vi "oax_Config TIO and DSA Channel (Single Shot).vi"(0 "master":T1={"DSA Device"="", "Channels"={"enable ch0"=FALSE, "enable ch1"=FALSE, "enable ch2"=FALSE, "enable ch3"=FALSE, "enable ch4"=FALSE, "enable ch5"=FALSE, "enable ch6"=FALSE, "enable ch7"=FALSE}, "Channel Names"={"ch0 string"="", "ch1 string"="", "ch2 string"="", "ch3 string"="", "ch4 string"="", "ch5 string"="", "ch6 string"="", "ch7 string"=""}, "Coupling"={"coupling ch0"=FALSE, "coupling ch1"=FALSE, "coupling ch2"=FALSE, "coupling ch3"=FALSE, "coupling ch4"=FALSE, "coupling ch5"=FALSE, "coupling ch6"=FALSE, "coupling ch7"=FALSE}, "IEPE"={"ICP ch0"=FALSE, "ICP ch0"=FALSE, "ICP ch0"=FALSE, "ICP ch0"=FALSE, "ICP ch0"=FALSE, "ICP ch0"=FALSE, "ICP ch0"=FALSE, "ICP ch0"=FALSE}, "Ch. Sensitivity\n[mV/EU]"={"ch0 sensitivity"=1000.0, "ch1 sensitivity"=1000.0, "ch2 sensitivity"=1000.0, "ch3 sensitivity"=1000.0, "ch4 sensitivity"=1000.0, "ch5 sensitivity"=1000.0, "ch6 sensitivity"=1000.0, "ch7 sensitivity"=1000.0}, "Engineering\nUnits"={"Engineering\nUnits"=0, "Engineering\nUnits"=0, "Engineering\nUnits"=0, "Engineering\nUnits"=0, "Engineering\nUnits"=0, "Engineering\nUnits"=0, "Engineering\nUnits"=0, "Engineering\nUnits"=0}, "Custom\nLabel"={"Custom Label"="", "Custom Label"="", "Custom Label"="", "Custom Label"="", "Custom Label"="", "Custom Label"="", "Custom Label"="", "Custom Label"=""}, "dB reference\n[EU]"={"dB reference [EU]"=1.0, "dB reference [EU]"=1.0, "dB reference [EU]"=1.0, "dB reference [EU]"=1.0, "dB reference [EU]"=1.0, "dB reference [EU]"=1.0, "dB reference [EU]"=1.0, "dB reference [EU]"=1.0}, "pregain\n[dB]"={"pregain [dB]"=0.0, "pregain [dB]"=0.0, "pregain [dB]"=0.0, "pregain [dB]"=0.0, "pregain [dB]"=0.0, "pregain [dB]"=0.0, "pregain [dB]"=0.0, "pregain [dB]"=0.0}, "Weighting\nFilter"={"Weighting Filter"=0, "Weighting Filter"=0, "Weighting Filter"=0, "Weighting Filter"=0, "Weighting Filter"=0, "Weighting Filter"=0, "Weighting Filter"=0, "Weighting Filter"=0}, "max value"=10.0, "min value"=0.0, "enable EAR?"=FALSE} {"min value" format="%0.2f"; "max value" format="%0.2f"; "Weighting\nFilter"."Weighting Filter" items=["Linear", "A-weighting", "B-weighting", "C-weighting", "ITU-R 468-4", "Dolby", "CCITT", "C-message"]; "Weighting\nFilter"."Weighting Filter" items=["Linear", "A-weighting", "B-weighting", "C-weighting", "ITU-R 468-4", "Dolby", "CCITT", "C-message"]; "Weighting\nFilter"."Weighting Filter" items=["Linear", "A-weighting", "B-weighting", "C-weighting", "ITU-R 468-4", "Dolby", "CCITT", "C-message"]; "Weighting\nFilter"."Weighting Filter" items=["Linear", "A-weighting", "B-weighting", "C-weighting", "ITU-R 468-4", "Dolby", "CCITT", "C-message"]; "Weighting\nFilter"."Weighting Filter" items=["Linear", "A-weighting", "B-weighting", "C-weighting", "ITU-R 468-4", "Dolby", "CCITT", "C-message"]; "Weighting\nFilter"."Weighting Filter" items=["Linear", "A-weighting", "B-weighting", "C-weighting", "ITU-R 468-4", "Dolby", "CCITT", "C-message"]; "Weighting\nFilter"."Weighting Filter" items=["Linear", "A-weighting", "B-weighting", "C-weighting", "ITU-R 468-4", "Dolby", "CCITT", "C-message"]; "Weighting\nFilter"."Weighting Filter" items=["Linear", "A-weighting", "B-weighting", "C-weighting", "ITU-R 468-4", "Dolby", "CCITT", "C-message"]; "pregain\n[dB]"."pregain [dB]" format="%.2f"; "pregain\n[dB]"."pregain [dB]" format="%.2f"; "pregain\n[dB]"."pregain [dB]" format="%.2f"; "pregain\n[dB]"."pregain [dB]" format="%.2f"; "pregain\n[dB]"."pregain [dB]" format="%.2f"; "pregain\n[dB]"."pregain [dB]" format="%.2f"; "pregain\n[dB]"."pregain [dB]" format="%.2f"; "pregain\n[dB]"."pregain [dB]" format="%.2f"; "dB reference\n[EU]"."dB reference [EU]" format="%^.1e"; "dB reference\n[EU]"."dB reference [EU]" format="%^.1e"; "dB reference\n[EU]"."dB reference [EU]" format="%^.1e"; "dB reference\n[EU]"."dB reference [EU]" format="%^.1e"; "dB reference\n[EU]"."dB reference [EU]" format="%^.1e"; "dB reference\n[EU]"."dB reference [EU]" format="%^.1e"; "dB reference\n[EU]"."dB reference [EU]" format="%^.1e"; "dB reference\n[EU]"."dB reference [EU]" format="%^.1e"; "Engineering\nUnits"."Engineering\nUnits" items=["custom..."=0, "V"=1, "A"=21, "Pa"=2, "N"=20, "g"=3, "m/s^2"=4, "m/s"=5, "m"=6, "mm/s"=12, "mm"=13, "microns/s"=14, "microns"=15, "in/s^2"=7, "in/s"=8, "in"=9, "mils/s"=10, "mils"=11, "rad/s^2"=16, "rad/s"=17, "rad"=18, "strain"=19]; "Engineering\nUnits"."Engineering\nUnits" items=["custom..."=0, "V"=1, "A"=21, "Pa"=2, "N"=20, "g"=3, "m/s^2"=4, "m/s"=5, "m"=6, "mm/s"=12, "mm"=13, "microns/s"=14, "microns"=15, "in/s^2"=7, "in/s"=8, "in"=9, "mils/s"=10, "mils"=11, "rad/s^2"=16, "rad/s"=17, "rad"=18, "strain"=19]; "Engineering\nUnits"."Engineering\nUnits" items=["custom..."=0, "V"=1, "A"=21, "Pa"=2, "N"=20, "g"=3, "m/s^2"=4, "m/s"=5, "m"=6, "mm/s"=12, "mm"=13, "microns/s"=14, "microns"=15, "in/s^2"=7, "in/s"=8, "in"=9, "mils/s"=10, "mils"=11, "rad/s^2"=16, "rad/s"=17, "rad"=18, "strain"=19]; "Engineering\nUnits"."Engineering\nUnits" items=["custom..."=0, "V"=1, "A"=21, "Pa"=2, "N"=20, "g"=3, "m/s^2"=4, "m/s"=5, "m"=6, "mm/s"=12, "mm"=13, "microns/s"=14, "microns"=15, "in/s^2"=7, "in/s"=8, "in"=9, "mils/s"=10, "mils"=11, "rad/s^2"=16, "rad/s"=17, "rad"=18, "strain"=19]; "Engineering\nUnits"."Engineering\nUnits" items=["custom..."=0, "V"=1, "A"=21, "Pa"=2, "N"=20, "g"=3, "m/s^2"=4, "m/s"=5, "m"=6, "mm/s"=12, "mm"=13, "microns/s"=14, "microns"=15, "in/s^2"=7, "in/s"=8, "in"=9, "mils/s"=10, "mils"=11, "rad/s^2"=16, "rad/s"=17, "rad"=18, "strain"=19]; "Engineering\nUnits"."Engineering\nUnits" items=["custom..."=0, "V"=1, "A"=21, "Pa"=2, "N"=20, "g"=3, "m/s^2"=4, "m/s"=5, "m"=6, "mm/s"=12, "mm"=13, "microns/s"=14, "microns"=15, "in/s^2"=7, "in/s"=8, "in"=9, "mils/s"=10, "mils"=11, "rad/s^2"=16, "rad/s"=17, "rad"=18, "strain"=19]; "Engineering\nUnits"."Engineering\nUnits" items=["custom..."=0, "V"=1, "A"=21, "Pa"=2, "N"=20, "g"=3, "m/s^2"=4, "m/s"=5, "m"=6, "mm/s"=12, "mm"=13, "microns/s"=14, "microns"=15, "in/s^2"=7, "in/s"=8, "in"=9, "mils/s"=10, "mils"=11, "rad/s^2"=16, "rad/s"=17, "rad"=18, "strain"=19]; "Engineering\nUnits"."Engineering\nUnits" items=["custom..."=0, "V"=1, "A"=21, "Pa"=2, "N"=20, "g"=3, "m/s^2"=4, "m/s"=5, "m"=6, "mm/s"=12, "mm"=13, "microns/s"=14, "microns"=15, "in/s^2"=7, "in/s"=8, "in"=9, "mils/s"=10, "mils"=11, "rad/s^2"=16, "rad/s"=17, "rad"=18, "strain"=19]; "Ch. Sensitivity\n[mV/EU]"."ch7 sensitivity" format="%.2f"; "Ch. Sensitivity\n[mV/EU]"."ch6 sensitivity" format="%.2f"; "Ch. Sensitivity\n[mV/EU]"."ch5 sensitivity" format="%.2f"; "Ch. Sensitivity\n[mV/EU]"."ch4 sensitivity" format="%.2f"; "Ch. Sensitivity\n[mV/EU]"."ch3 sensitivity" format="%.2f"; "Ch. Sensitivity\n[mV/EU]"."ch2 sensitivity" format="%.2f"; "Ch. Sensitivity\n[mV/EU]"."ch1 sensitivity" format="%.2f"; "Ch. Sensitivity\n[mV/EU]"."ch0 sensitivity" format="%.2f"}, 1 "samples per channel":u32, 2 "sample rate [samples/s]":dbl, 5 "Counter(s)":tag, 9 "PFI line (Gate)":tag, 11 "error out":errorcluster, 12 "Tacho Pulse Edge":i32, 13 "Slave Slot Number":i32(ring) caption="PXI Slot Number" items=["Slot 3", "Slot 4", "Slot 5", "Slot 6", "Slot 7", "Slot 8", "Slot 9", "Slot 10", "Slot 11", "Slot 12", "Slot 13", "Slot 14", "Slot 15", "Slot 16"], 14 "DSA device type":u16(ring) items=["447x", "446x"]) -> (4 "DSA task out":refnum<k21>, 6 "TIO task out":refnum<k21>, 15 "error in":errorcluster)   [LabVIEW 2017]
doc: "Configures DAQ channel properties based on the user input and starts the DAQmx task."
uses:
  <vilib>/addons/Sound and Vibration/Order Analysis/Example Support/sub VIs/OAXML_Analog Channel Config (DAQmx).ctl
  <vilib>/DAQmx/configure/timing.llb/DAQmx Timing (Sample Clock).vi
  <vilib>/DAQmx/create/channels.llb/DAQmx Create Channel (CI-Count Edges).vi
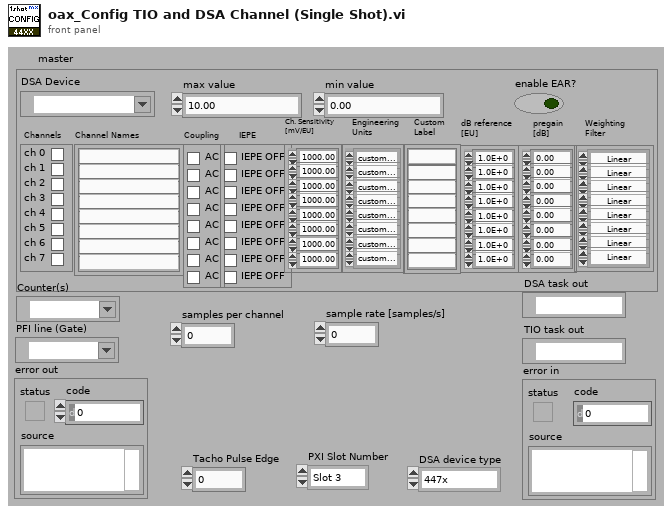
[diagram p1: front panel]
types:
  T1 = typedef "OAXML_Analog Channel Config (DAQmx).ctl" = cluster{"DSA Device":tag, "Channels":cluster{"enable ch0":bool, "enable ch1":bool, "enable ch2":bool, "enable ch3":bool, "enable ch4":bool, "enable ch5":bool, "enable ch6":bool, "enable ch7":bool}, "Channel Names":cluster{"ch0 string":string, "ch1 string":string, "ch2 string":string, "ch3 string":string, "ch4 string":string, "ch5 string":string, "ch6 string":string, "ch7 string":string}, "Coupling":cluster{"coupling ch0":bool, "coupling ch1":bool, "coupling ch2":bool, "coupling ch3":bool, "coupling ch4":bool, "coupling ch5":bool, "coupling ch6":bool, "coupling ch7":bool}, "IEPE":cluster{"ICP ch0":bool, "ICP ch0":bool, "ICP ch0":bool, "ICP ch0":bool, "ICP ch0":bool, "ICP ch0":bool, "ICP ch0":bool, "ICP ch0":bool}, "Ch. Sensitivity\n[mV/EU]":cluster{"ch0 sensitivity":dbl, "ch1 sensitivity":dbl, "ch2 sensitivity":dbl, "ch3 sensitivity":dbl, "ch4 sensitivity":dbl, "ch5 sensitivity":dbl, "ch6 sensitivity":dbl, "ch7 sensitivity":dbl}, "Engineering\nUnits":cluster{"Engineering\nUnits":u16, "Engineering\nUnits":u16, "Engineering\nUnits":u16, "Engineering\nUnits":u16, "Engineering\nUnits":u16, "Engineering\nUnits":u16, "Engineering\nUnits":u16, "Engineering\nUnits":u16}, "Custom\nLabel":cluster{"Custom Label":string, "Custom Label":string, "Custom Label":string, "Custom Label":string, "Custom Label":string, "Custom Label":string, "Custom Label":string, "Custom Label":string}, "dB reference\n[EU]":cluster{"dB reference [EU]":dbl, "dB reference [EU]":dbl, "dB reference [EU]":dbl, "dB reference [EU]":dbl, "dB reference [EU]":dbl, "dB reference [EU]":dbl, "dB reference [EU]":dbl, "dB reference [EU]":dbl}, "pregain\n[dB]":cluster{"pregain [dB]":dbl, "pregain [dB]":dbl, "pregain [dB]":dbl, "pregain [dB]":dbl, "pregain [dB]":dbl, "pregain [dB]":dbl, "pregain [dB]":dbl, "pregain [dB]":dbl}, "Weighting\nFilter":cluster{"Weighting Filter":u16, "Weighting Filter":u16, "Weighting Filter":u16, "Weighting Filter":u16, "Weighting Filter":u16, "Weighting Filter":u16, "Weighting Filter":u16, "Weighting Filter":u16}, "max value":dbl, "min value":dbl, "enable EAR?":bool}
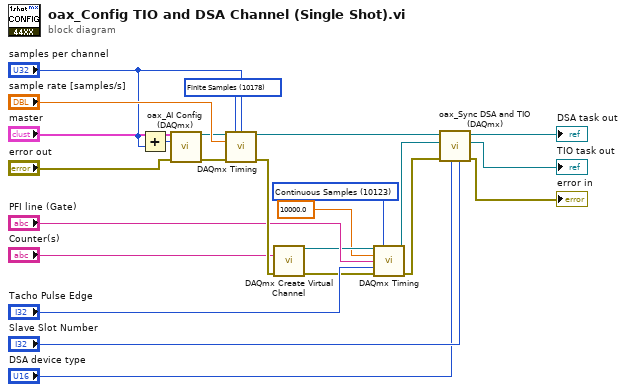
[diagram p0: block diagram]
diagram:
  w9 = 10123 items=["Finite Samples"=10178, "Continuous Samples"=10123, "Hardware Timed Single Point"=12522] ("sample mode")
  w8 = 10178 items=["Finite Samples"=10178, "Continuous Samples"=10123, "Hardware Timed Single Point"=12522] ("sample mode")
  n1 = Add(x="samples per channel", y="samples per channel") -> (x+y=w3:u32)
  n2 = call <vilib>:"oax_AI Config (DAQmx).vi"("master"="master", "buffer size"=w3, "error in (no error)"="error out") -> ("task out"=w6:refnum<k21>, "error out"=w7:errorcluster)  [unwired: 11 in]
  n3 = call-poly <vilib>:"DAQmx Timing.vi"("task/channels in"=w6, "sample mode"=w8, "samples per channel"="samples per channel", "rate"="sample rate [samples/s]", "error in"=w7) -> ("task out"=w21:refnum<k21>, "error out"=w24:errorcluster)  [unwired: 9 in]
  n4 = call-poly <vilib>:"DAQmx Create Virtual Channel.vi"("counter"="Counter(s)", "error in"=w24) -> ("task out"=w13:refnum<k21>, "error out"=w14:errorcluster)  [unwired: 12 in]
  n5 = call-poly <vilib>:"DAQmx Timing.vi"("task/channels in"=w13, "sample mode"=w9, "rate"=10000.0, "source"="PFI line (Gate)", "active edge"="Tacho Pulse Edge", "error in"=w14) -> ("task out"=w15:refnum<k21>, "error out"=w16:errorcluster)  [unwired: 8 in]
  n6 = call <vilib>:"oax_Sync DSA and TIO (DAQmx).vi"("Slave Slot Number"="Slave Slot Number", "DSA device type"="DSA device type", "error in"=w16, "TIO task in"=w15, "DSA task in"=w21) -> ("error in"=→"error in":errorcluster, "TIO task out"=→"TIO task out":refnum<k21>, "DSA task out"=→"DSA task out":refnum<k21>)  [unwired: 4 in]
